vi "Execution End.vi"(8 "error in (no error)":errorcluster, 10 "Execution in":refnum<data-value>, 11 "Plugin in":refnum<class "Plugin.lvclass">) -> (0 "error out":errorcluster, 2 "Execution out":refnum<data-value>, 3 "Plugin out":refnum<class "Plugin.lvclass">)   [LabVIEW 2015, in "Plugin.lvclass"]
uses:
  Plugin.lvclass
  Execution.lvclass
  Step.lvclass
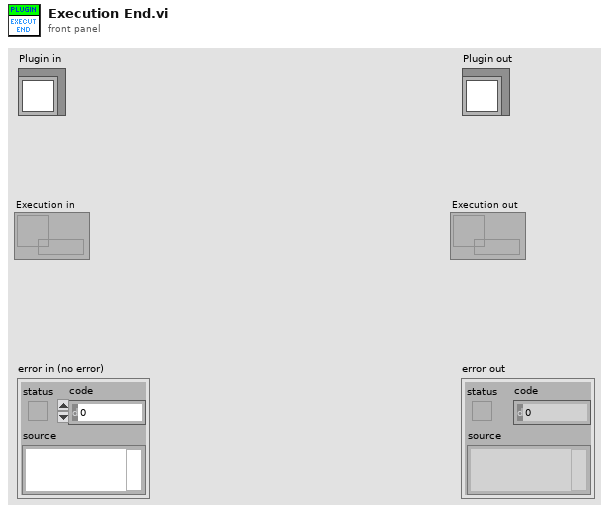
[diagram p1: front panel]
types:
  T1 = typedef "Execution.lvclass/STEP_CONTEXT.ctl" = cluster{"StepIndex":u32, "Step":refnum<class "Step.lvclass">, "StartTime":timestamp, "EndTime":timestamp, "Result":T2, "Error Info":string, "Output Values":cluster{"Name":string, "Variant Data":variant}[]}
  T2 = typedef "Step.lvclass/STEP_STATUS.ctl" = enum16{"Skipped", "Done", "Passed", "Failed", "Error"}
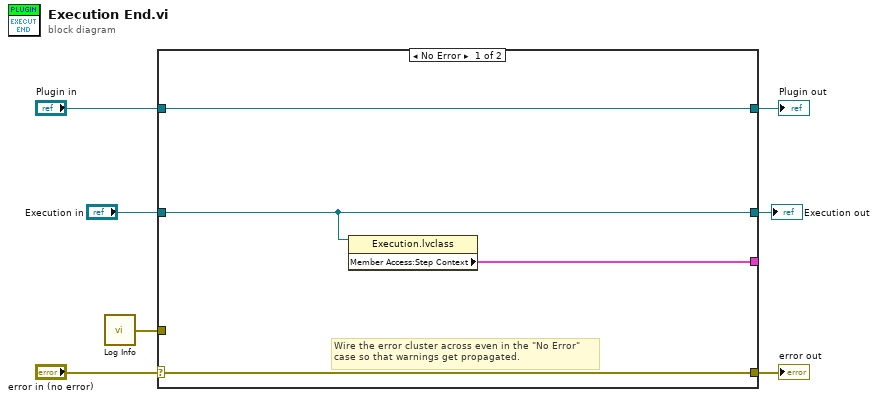
[diagram p0: block diagram]
diagram:
  n1 = call "Log Info.vi"() -> ("error out"=w1:errorcluster)  [unwired: 5 in]
  n2 = case shown="No Error" "error in (no error)" {
    selector: "error in (no error)" -> [w10 w14]
    tunnel: [w10 w14] -> w6
    tunnel: [w11 w13] -> w4
    tunnel: "Plugin in" -> [w11 w13]
    tunnel: "Execution in" -> [w9 w12]
    tunnel: [w9 w12] -> w2
    tunnel: w1 -> [_ _]
    tunnel: [w8 _] -> _
    frame No Error {
      # "Wire the error cluster across even in the \"No Error\"\ncase so that warnings get propagated."
      n3 = property class="Execution.lvclass"(reference=w9) -> ("Member Access:Step Context"=w8:T1)  [unwired: 1 in, 2 out]
    }
    frame Error {
    }
  }
  "error out" <- w6
  "Plugin out" <- w4
  "Execution out" <- w2
